vi "Take uWave Reading.vi"(8 "error in (no error)":errorcluster, 10 "H3611i":bool, 11 "MWWL Verification in":refnum<class "MWWL Verification.lvclass">) -> (0 "error out":errorcluster, 3 "MWWL Verification out":refnum<class "MWWL Verification.lvclass">)   [LabVIEW 2017, in "MWWL Verification.lvlib" / "MWWL Verification.lvclass"]
uses:
  MWWL Verification.lvclass
  H3611i Actor/H3611i Actor Messages/Measure H3611i Range Msg/Measure H3611i Range Msg.lvclass
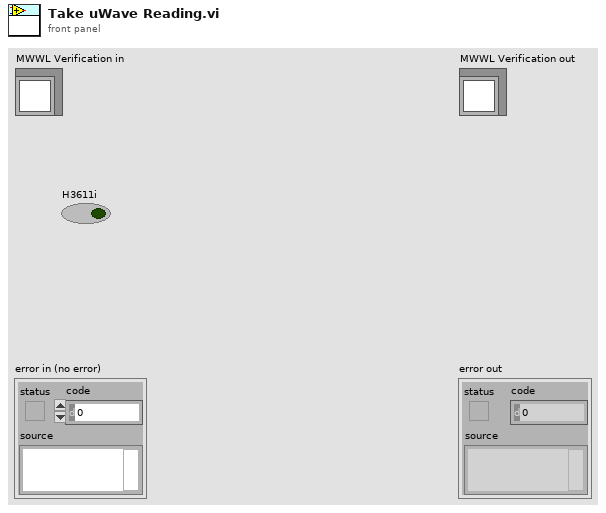
[diagram p1: front panel]
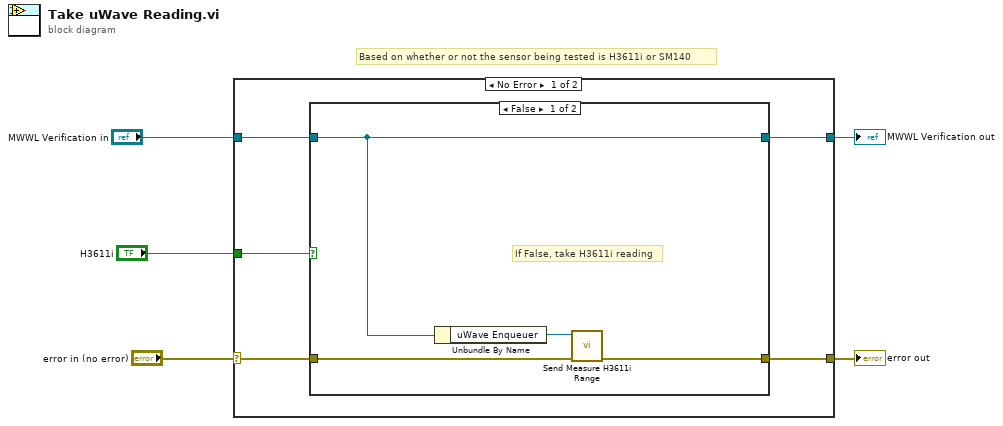
[diagram p0: block diagram]
diagram:
  # "Based on whether or not the sensor being tested is H3611i or SM140"
  n1 = case shown="No Error" "error in (no error)" {
    selector: "error in (no error)" -> [w7 w18]
    tunnel: [w6 w18] -> w4
    tunnel: [w8 w17] -> w2
    tunnel: "MWWL Verification in" -> [w9 w17]
    tunnel: "H3611i" -> [w10 _]
    frame No Error {
      n2 = case shown="False" w10 {
        tunnel: w9 -> [w14 w16]
        tunnel: [w14 w16] -> w8
        tunnel: w7 -> [w12 w15]
        tunnel: [w11 w15] -> w6
        frame False {
          # "If False, take H3611i reading"
          n3 = Unbundle By Name(w14) -> ("uWave Enqueuer"=w13:refnum<class "Message Enqueuer.lvclass">)
          n4 = call "Send Measure H3611i Range.vi"("error in (no error)"=w12, "Message Enqueuer in"=w13) -> ("error out"=w11:errorcluster)  [unwired: 8 in, 1 out]
        }
        frame True {
        }
      }
    }
    frame Error {
    }
  }
  "error out" <- w4
  "MWWL Verification out" <- w2
